vi "Folder exists.vi"(11 "path":path) -> (3 "folder exists?":bool)   [LabVIEW 2012]
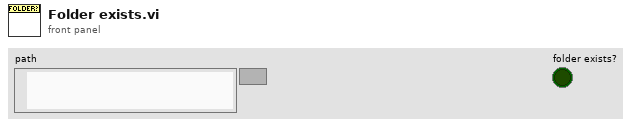
[diagram p1: front panel]
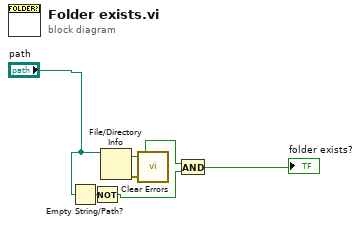
[diagram p0: block diagram]
diagram:
  n1 = Empty String/Path?(string/path="path") -> (empty?=w5:bool)
  n2 = Not(x=w5) -> (.not. x?=w3:bool)
  n3 = File/Directory Info(path="path") -> (directory=w4:bool, error out=w1:errorcluster)  [unwired: 1 in, 5 out]
  n4 = call <vilib>:"Clear Errors.vi"("error in (no error)"=w1) -> ()  [unwired: 6 in, 1 out]
  n5 = And(x=w4, y=w3) -> (x .and. y?=→"folder exists?":bool)
